vi "BuildTag.vi"(0 "Indent":i8=-1, 2 "tag":string, 3 "value":string, 4 "string in":string) -> (1 "string out":string)   [LabVIEW 2013]
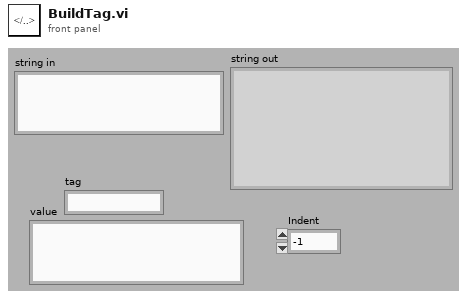
[diagram p1: front panel]
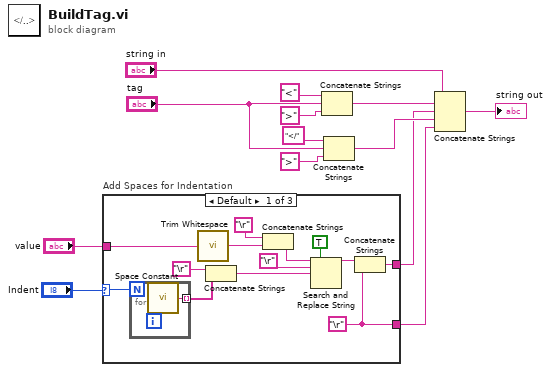
[diagram p0: block diagram]
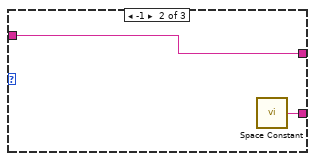
[diagram p2: hidden frame]
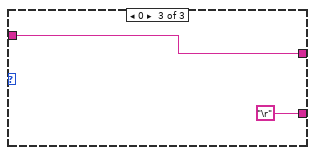
[diagram p3: hidden frame]
diagram:
  n1 = case "Add Spaces for Indentation" shown="Default" "Indent" {
    selector: "Indent" -> [w16 _ _]
    tunnel: [w24 w29 w31] -> w5
    tunnel: "value" -> [w21 w29 w31]
    tunnel: [w14 w28 "\r"] -> w1
    frame Default {
      w14 = "\r"
      n2 = for {
        N: w16 -> [_]
        tunnel: [w27] -> w18 mode=indexing
        n3 = call <vilib>:"Space Constant.vi"() -> ("String"=w27:string)
      }
      n4 = call <vilib>:"Trim Whitespace.vi"("string"=w21) -> ("trimmed string"=w20:string)  [unwired: 1 in]
      n5 = Concatenate Strings("\r", w18) -> (w17:string)
      n6 = Concatenate Strings("\r", w20) -> (w22:string)
      n7 = Search and Replace String(replace all?=TRUE ("replace all? (F)"), input string=w22, search string="\r", replace string=w17) -> (result string=w25:string)  [unwired: 4 in, 3 out]
      n8 = Concatenate Strings(w25, w14) -> (w24:string)
    }
    frame -1 {
      n9 = call <vilib>:"Space Constant.vi"() -> ("String"=w28:string)
    }
    frame 0 {
    }
  }
  n10 = Concatenate Strings("<", "tag", ">") -> (w11:string)
  n11 = Concatenate Strings("</", "tag", ">") -> (w12:string)
  n12 = Concatenate Strings("string in", w11, w5, w12, w1) -> (→"string out":string)
